vi "Sub_Online_FFT_Main.vi"(9 "Bound to 1st Frequency":bool=TRUE, 10 "Frequency Method":T3(ring), 11 "Experiment in":T1) -> (2 "looping":bool, 3 "Experiment out":T2)   [LabVIEW 2021]
uses:
  Desktop/VI's/HIL WORKING/Control 1.ctl
panel:
  out "Low-Energy Warning":bool
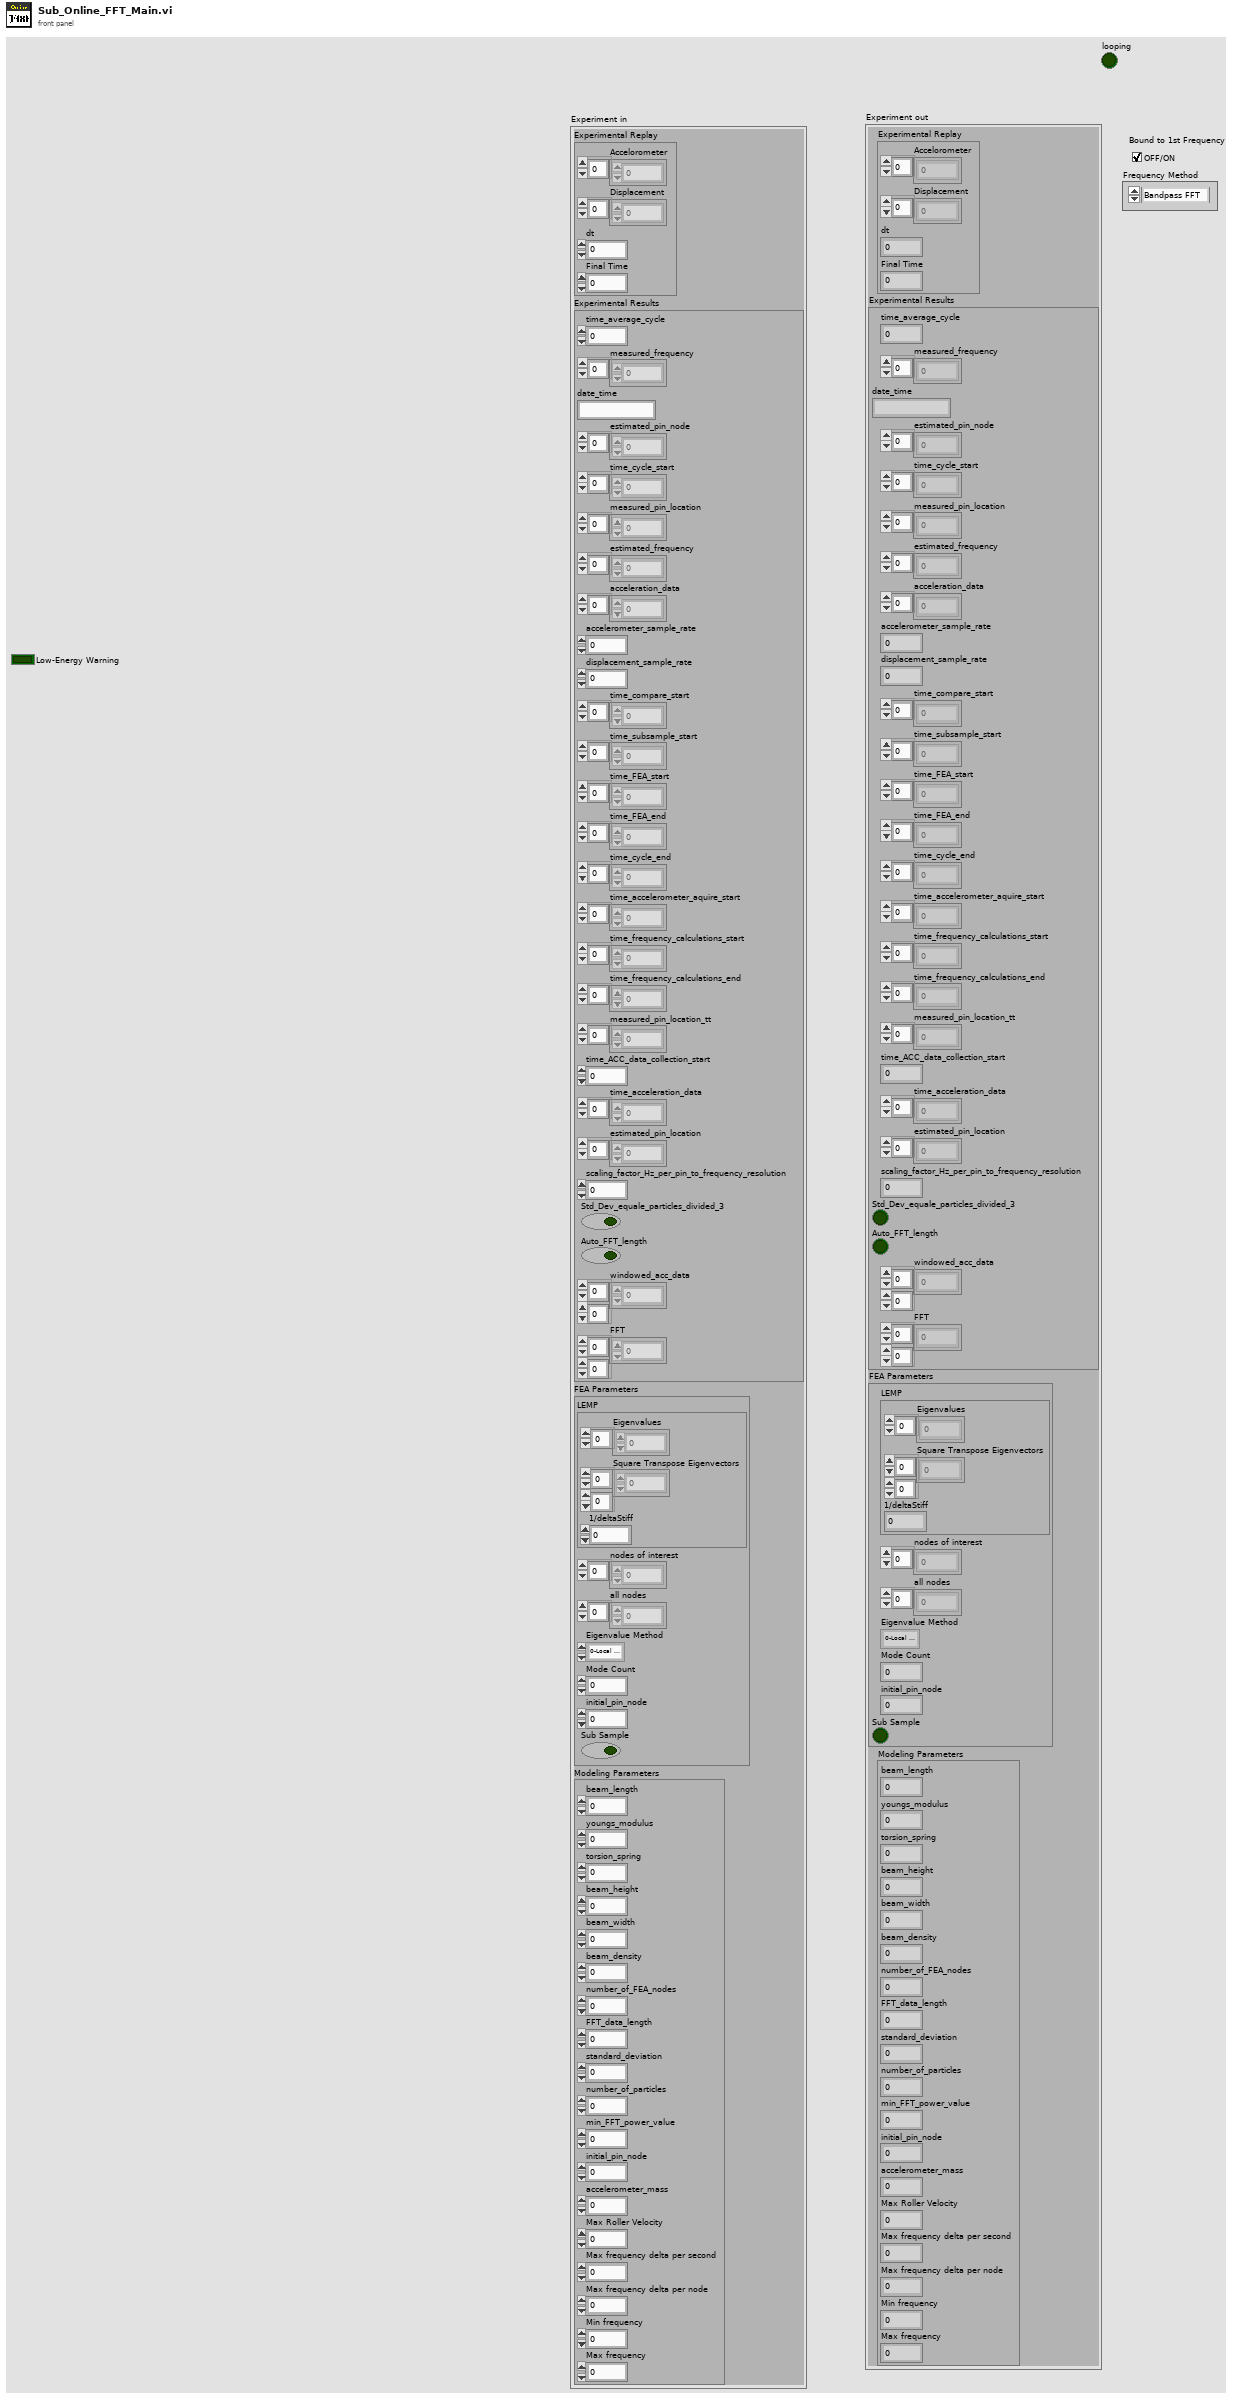
[diagram p1: front panel]
types:
  T1 = cluster{"Experimental Replay":cluster{"Accelorometer":dbl[], "Displacement":dbl[], "dt":dbl, "Final Time":dbl}, "Experimental Results":cluster{"time_average_cycle":dbl, "measured_frequency":dbl[], "date_time":string, "estimated_pin_node":i32[], "time_cycle_start":dbl[], "measured_pin_location":dbl[], "estimated_frequency":dbl[], "acceleration_data":dbl[], "accelerometer_sample_rate":dbl, "displacement_sample_rate":dbl, "time_compare_start":dbl[], "time_subsample_start":dbl[], "time_FEA_start":dbl[], "time_FEA_end":dbl[], "time_cycle_end":dbl[], "time_accelerometer_aquire_start":dbl[], "time_frequency_calculations_start":dbl[], "time_frequency_calculations_end":dbl[], "measured_pin_location_tt":dbl[], "time_ACC_data_collection_start":dbl, "time_acceleration_data":dbl[], "estimated_pin_location":dbl[], "scaling_factor_Hz_per_pin_to_frequency_resolution":dbl, "Std_Dev_equale_particles_divided_3":bool, "Auto_FFT_length":bool, "windowed_acc_data":dbl[][], "FFT":dbl[][]}, "FEA Parameters":cluster{"LEMP":cluster{"Eigenvalues":dbl[], "Square Transpose Eigenvectors":dbl[][], "1/deltaStiff":dbl}, "nodes of interest":i32[], "all nodes":i32[], "Eigenvalue Method":enum16{"0-Local Eigen Modification Procedure", "1-LabVIEW generalized eigenvalues", "2-LabVIEW M^-1K eigenvalues", "3-LabVIEW Cholesky Factorization", "4-Cholesky Factorization CPU SGL", "5-Cholesky Factorization CPU FXP", "6-Cholesky Factorization FPGA SGL", "7-Cholesky Factorization FPGA SGL SCL"}, "Mode Count":i32, "initial_pin_node":i32, "Sub Sample":bool}, "Modeling Parameters":cluster{"beam_length":dbl, "youngs_modulus":dbl, "torsion_spring":dbl, "beam_height":dbl, "beam_width":dbl, "beam_density":dbl, "number_of_FEA_nodes":i32, "FFT_data_length":i32, "standard_deviation":dbl, "number_of_particles":i32, "min_FFT_power_value":dbl, "initial_pin_node":i32, "accelerometer_mass":dbl, "Max Roller Velocity":dbl, "Max frequency delta per second":dbl, "Max frequency delta per node":dbl, "Min frequency":dbl, "Max frequency":dbl}}
  T2 = typedef "Control 1.ctl" = cluster{"Experimental Replay":cluster{"Accelorometer":dbl[], "Displacement":dbl[], "dt":dbl, "Final Time":dbl}, "Experimental Results":cluster{"time_average_cycle":dbl, "measured_frequency":dbl[], "date_time":string, "estimated_pin_node":i32[], "time_cycle_start":dbl[], "measured_pin_location":dbl[], "estimated_frequency":dbl[], "acceleration_data":dbl[], "accelerometer_sample_rate":dbl, "displacement_sample_rate":dbl, "time_compare_start":dbl[], "time_subsample_start":dbl[], "time_FEA_start":dbl[], "time_FEA_end":dbl[], "time_cycle_end":dbl[], "time_accelerometer_aquire_start":dbl[], "time_frequency_calculations_start":dbl[], "time_frequency_calculations_end":dbl[], "measured_pin_location_tt":dbl[], "time_ACC_data_collection_start":dbl, "time_acceleration_data":dbl[], "estimated_pin_location":dbl[], "scaling_factor_Hz_per_pin_to_frequency_resolution":dbl, "Std_Dev_equale_particles_divided_3":bool, "Auto_FFT_length":bool, "windowed_acc_data":dbl[][], "FFT":dbl[][]}, "FEA Parameters":cluster{"LEMP":cluster{"Eigenvalues":dbl[], "Square Transpose Eigenvectors":dbl[][], "1/deltaStiff":dbl}, "nodes of interest":i32[], "all nodes":i32[], "Eigenvalue Method":enum16{"0-Local Eigen Modification Procedure", "1-LabVIEW generalized eigenvalues", "2-LabVIEW M^-1K eigenvalues", "3-LabVIEW Cholesky Factorization", "4-Cholesky Factorization CPU SGL", "5-Cholesky Factorization CPU FXP", "6-Cholesky Factorization FPGA SGL", "7-Cholesky Factorization FPGA SGL SCL"}, "Mode Count":i32, "initial_pin_node":i32, "Sub Sample":bool}, "Modeling Parameters":cluster{"beam_length":dbl, "youngs_modulus":dbl, "torsion_spring":dbl, "beam_height":dbl, "beam_width":dbl, "beam_density":dbl, "number_of_FEA_nodes":i32, "FFT_data_length":i32, "standard_deviation":dbl, "number_of_particles":i32, "min_FFT_power_value":dbl, "initial_pin_node":i32, "accelerometer_mass":dbl, "Max Roller Velocity":dbl, "Max frequency delta per second":dbl, "Max frequency delta per node":dbl, "Min frequency":dbl, "Max frequency":dbl}}
  T3 = enum16{"Bandpass FFT", "Tone", "FFT", "Custom Filter"}
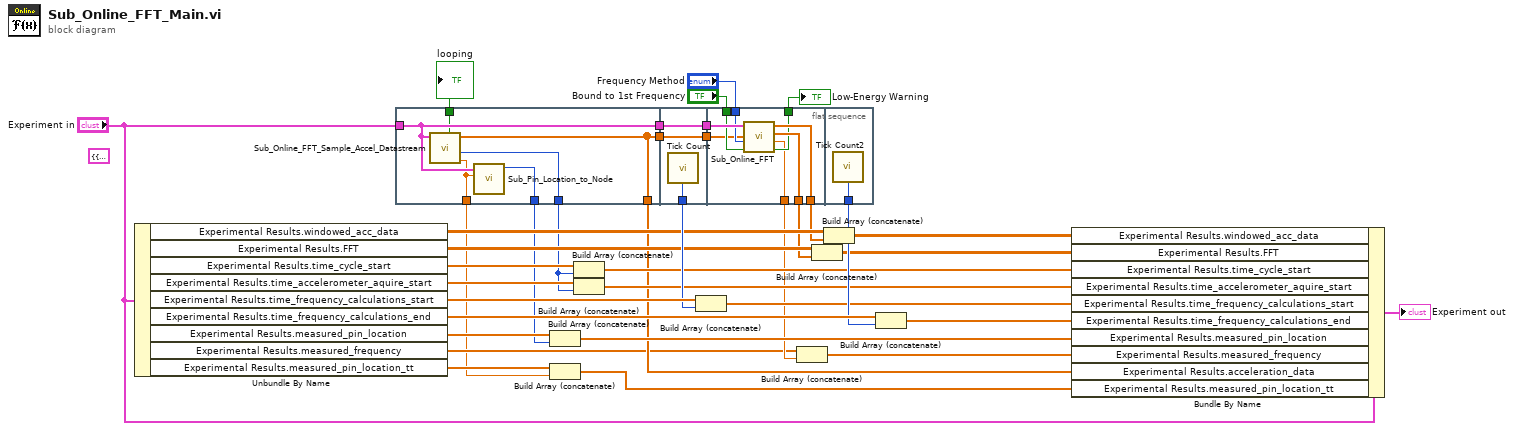
[diagram p0: block diagram]
diagram:
  (unwired) T1 {"Experimental Replay"={"Accelorometer"=[], "Displacement"=[], "dt"=0.0, "Final Time"=0.0}, "Experimental Results"={"time_average_cycle"=0.0, "measured_frequency"=[], "date_time"="", "estimated_pin_node"=[], "time_cycle_start"=[], "measured_pin_location"=[], "estimated_frequency"=[], "acceleration_data"=[], "accelerometer_sample_rate"=0.0, "displacement_sample_rate"=0.0, "time_compare_start"=[], "time_subsample_start"=[], "time_FEA_start"=[], "time_FEA_end"=[], "time_cycle_end"=[], "time_accelerometer_aquire_start"=[], "time_frequency_calculations_start"=[], "time_frequency_calculations_end"=[], "measured_pin_location_tt"=[], "time_ACC_data_collection_start"=0.0, "time_acceleration_data"=[], "estimated_pin_location"=[], "scaling_factor_Hz_per_pin_to_frequency_resolution"=0.0, "Std_Dev_equale_particles_divided_3"=FALSE, "Auto_FFT_length"=FALSE, "windowed_acc_data"=[], "FFT"=[]}, "FEA Parameters"={"LEMP"={"Eigenvalues"=[], "Square Transpose Eigenvectors"=[], "1/deltaStiff"=0.0}, "nodes of interest"=[], "all nodes"=[], "Eigenvalue Method"=enum."0-Local Eigen Modification Procedure", "Mode Count"=0, "initial_pin_node"=0, "Sub Sample"=FALSE}, "Modeling Parameters"={"beam_length"=0.0, "youngs_modulus"=0.0, "torsion_spring"=0.0, "beam_height"=0.0, "beam_width"=0.0, "beam_density"=0.0, "number_of_FEA_nodes"=0, "FFT_data_length"=0, "standard_deviation"=0.0, "number_of_particles"=0, "min_FFT_power_value"=0.0, "initial_pin_node"=0, "accelerometer_mass"=0.0, "Max Roller Velocity"=0.0, "Max frequency delta per second"=0.0, "Max frequency delta per node"=0.0, "Min frequency"=0.0, "Max frequency"=0.0}} ("Experiment")
  n1 = Unbundle By Name("Experiment in") -> ("Experimental Results.windowed_acc_data"=w22:dbl[][], "Experimental Results.FFT"=w20:dbl[][], "Experimental Results.time_cycle_start"=w28:dbl[], "Experimental Results.time_accelerometer_aquire_start"=w27:dbl[], "Experimental Results.time_frequency_calculations_start"=w31:dbl[], "Experimental Results.time_frequency_calculations_end"=w35:dbl[], "Experimental Results.measured_pin_location"=w29:dbl[], "Experimental Results.measured_frequency"=w6:dbl[], "Experimental Results.measured_pin_location_tt"=w5:dbl[])
  n2 = flat-sequence {
    tunnel: [w40] -> w37
    tunnel: [w43] -> w3
    tunnel: "Experiment in" -> [w41]
    tunnel: [w42] -> w15
    tunnel: [w41] -> w12
    tunnel: [w40] -> w10
    tunnel: [w39] -> w2
    tunnel: [w38] -> w1
    tunnel: w37 -> [w46]
    tunnel: [w46] -> w36
    tunnel: [w45] -> w30
    tunnel: w12 -> [w44]
    tunnel: [w44] -> w11
    tunnel: w36 -> [w48]
    tunnel: [w53] -> w17
    tunnel: [w52] -> w18
    tunnel: [w47] -> w16
    tunnel: w11 -> [w54]
    tunnel: "Frequency Method" -> [w51]
    tunnel: [w50] -> w8
    tunnel: "Bound to 1st Frequency" -> [w49]
    tunnel: [w55] -> w34
    frame #0 {
      n3 = call "Sub_Online_FFT_Sample_Accel_Datastream.vi"("Experiment"=w41) -> ("Last pin pos"=w39:dbl, "Sample Time"=w42:u32, "Accelerometer sample"=w40:dbl[], "looping"=w38:bool)  [unwired: 6 in, 1 out]
      n4 = call "Sub_Pin_Location_to_Node.vi"("Pin Location"=w39, "Experiment in"=w41) -> ("DOF of Interest"=w43:i32)  [unwired: 9 in]
    }
    frame #1 {
      n5 = call "Tick Count"() -> ("Tick Count(uSec)"=w45:u32)
    }
    frame #2 {
      n6 = call "Sub_Online_FFT.vi"("Bound to 1st Frequency"=w49, "Frequency Method"=w51, "Accelerometer sample"=w48, "Experiment"=w54) -> ("Low-Energy Warning"=w50:bool, "Frequency measured"=w47:dbl, "FFT"=w52:dbl[], "ACC Data"=w53:dbl[])  [unwired: 4 in]
    }
    frame #3 {
      n7 = call "Tick Count2"() -> ("Tick Count(uSec)"=w55:u32)
    }
  }
  n8 = Build Array (concatenate)(w29, w3) -> (w26:dbl[])
  n9 = Build Array (concatenate)(w5, w2) -> (w4:dbl[])
  n10 = Build Array (concatenate)(w28, w15) -> (w25:dbl[])
  n11 = Build Array (concatenate)(w27, w15) -> (w24:dbl[])
  n12 = Build Array (concatenate)(w31, w30) -> (w23:dbl[])
  n13 = Build Array (concatenate)(w6, w16) -> (w33:dbl[])
  n14 = Build Array (concatenate)(w20, w18) -> (w19:dbl[][])
  n15 = Build Array (concatenate)(w22, w17) -> (w21:dbl[][])
  n16 = Build Array (concatenate)(w35, w34) -> (w32:dbl[])
  n17 = Bundle By Name(cluster="Experiment in", "Experimental Results.windowed_acc_data"=w21, "Experimental Results.FFT"=w19, "Experimental Results.time_cycle_start"=w25, "Experimental Results.time_accelerometer_aquire_start"=w24, "Experimental Results.time_frequency_calculations_start"=w23, "Experimental Results.time_frequency_calculations_end"=w32, "Experimental Results.measured_pin_location"=w26, "Experimental Results.measured_frequency"=w33, "Experimental Results.acceleration_data"=w10, "Experimental Results.measured_pin_location_tt"=w4) -> (→"Experiment out":T1)
  "Low-Energy Warning" <- w8
  "looping" <- w1
